vi "tmp.vi"(11 "XYGraph Refnum":refnum<vi>) -> (2 "resulting string":string)   [LabVIEW 2014, in "Graph.lvclass"]
uses:
  Graph.lvclass
  <vilib>/Analysis/1siggen.llb/Ramp Pattern by Samples.vi
  <userlib>/_OpenG.lib/array/array.llb/Remove Duplicates from 1D Array (U32)__ogtk.vi
  <userlib>/_OpenG.lib/array/array.llb/Delete Elements from 1D Array (String)__ogtk.vi
  <vilib>/gmath/NI_Gmath.lvlib
  <vilib>/Analysis/NI_AALBase.lvlib
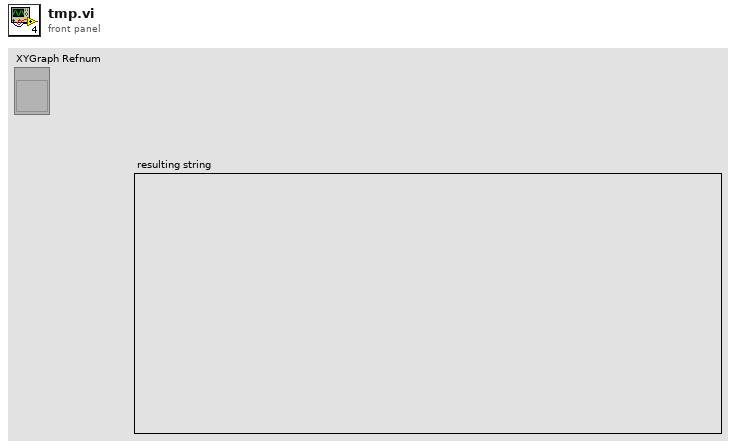
[diagram p1: front panel]
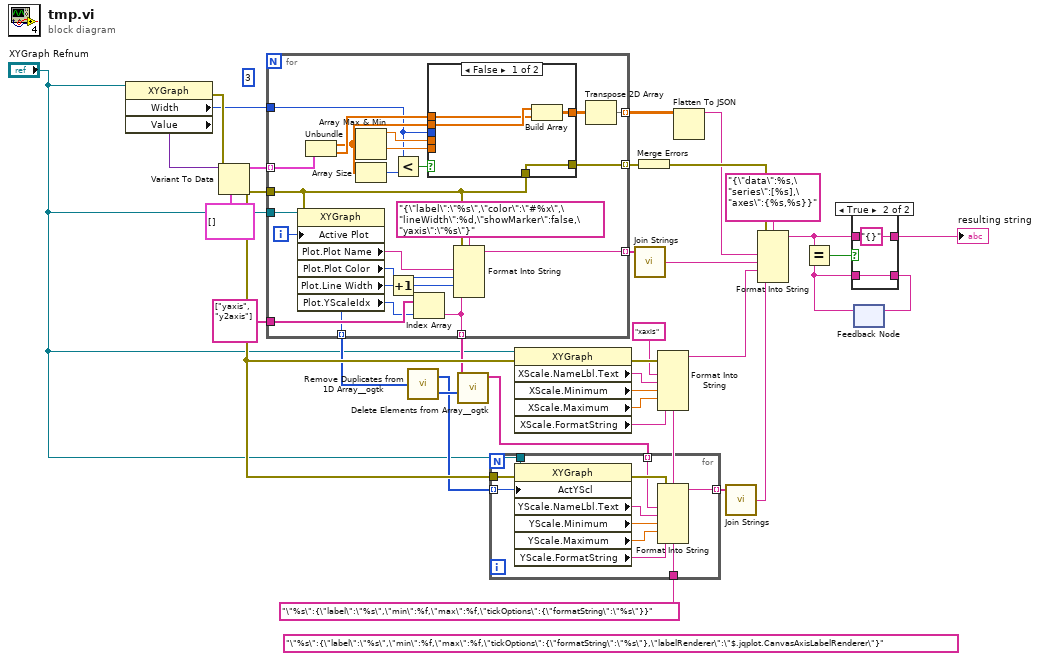
[diagram p0: block diagram]
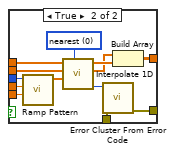
[diagram p3: hidden frame]
diagram:
  (unwired) "\"%s\":{\"label\":\"%s\",\"min\":%f,\"max\":%f,\"tickOptions\":{\"formatString\":\"%s\"},\"labelRenderer\":\"$.jqplot.CanvasAxisLabelRenderer\"}"
  (unwired) 3
  w7 = "\"%s\":{\"label\":\"%s\",\"min\":%f,\"max\":%f,\"tickOptions\":{\"formatString\":\"%s\"}}"
  n1 = property class="XYGraph"(reference="XYGraph Refnum") -> (error out=w35:errorcluster, "Width"=w6:u32, "Value"=w31:variant)  [unwired: 1 in, 1 out]
  n2 = Variant To Data(error in=w35, type=cluster{dbl[], dbl[]}[] [], Variant=w31) -> (data=w29:cluster{dbl[], dbl[]}[], error out=w34:errorcluster)
  n3 = for {
    tunnel: [w56] -> w9 mode=indexing
    tunnel: w29 -> [w53] mode=indexing
    tunnel: "XYGraph Refnum" -> [w40]
    tunnel: [w58] -> w28 mode=indexing
    tunnel: w6 -> [w47]
    tunnel: w34 -> [w57]
    tunnel: string[] ["yaxis", "y2axis"] -> [w41]
    tunnel: [w39] -> w13 mode=indexing
    tunnel: [w38] -> w12 mode=indexing
    tunnel: [w37] -> w11 mode=indexing
    i -> [w42]
    n4 = property on="Property Node" class="XYGraph"(reference=w40, error in=w57, "Active Plot"=w42) -> ("Plot.Plot Name"=w44:string, "Plot.Plot Color"=w45:u32, "Plot.Line Width"=w46:u8, "Plot.YScaleIdx"=w39:u32)  [unwired: 2 out]
    n5 = Unbundle(w53) -> (w49:dbl[], w54:dbl[])
    n6 = Array Max & Min(array=w49) -> (max value=w52:dbl, min value=w51:dbl)  [unwired: 2 out]
    n7 = Array Size(array=w49) -> (size(s)=w48:i32)
    n8 = Increment(x=w46) -> (x+1=w36:u8)
    n9 = Less?(x=w47, y=w48) -> (x < y?=w50:bool)
    n10 = Index Array(array=w41, index=w39) -> (element=w38:string)
    n11 = case shown="False" w50 {
      tunnel: [w59 w75] -> w58
      tunnel: [w62 w73] -> w55
      tunnel: w54 -> [w60 w72]
      tunnel: w49 -> [w61 w66]
      tunnel: w52 -> [_ w65]
      tunnel: w51 -> [_ w64]
      tunnel: w47 -> [_ w63]
      tunnel: w57 -> [w59 w74]
      frame False {
        n12 = Build Array(w61, w60) -> (w62:dbl[][])
      }
      frame True {
        w67 = 0 items=["nearest", "linear", "spline", "cubic Hermite", "Lagrange"] ("method")
        n13 = call-poly <vilib>:"Ramp Pattern.vi"("start"=w64, "end"=w65, "samples"=w63) -> ("Ramp Pattern"=w68:dbl[])  [unwired: 7 in, 1 out]
        n14 = call <vilib>:"Interpolate 1D.vi"("method"=w67, "xi"=w68, "X"=w66, "Y"=w72) -> ("error"=w69:i32, "xi used"=w70:dbl[], "yi"=w71:dbl[])  [unwired: 5 in]
        n15 = call <vilib>:"Error Cluster From Error Code.vi"("error in (no error)"=w74, "error code (0)"=w69) -> ("error out"=w75:errorcluster)  [unwired: 7 in]
        n16 = Build Array(w70, w71) -> (w73:dbl[][])
      }
    }
    n17 = Format Into String(format string="{\"label\":\"%s\",\"color\":\"#%x\",\"lineWidth\":%d,\"showMarker\":false,\"yaxis\":\"%s\"}", error in=w57, w44, w45, w36, w38) -> (resulting string=w37:string)  [unwired: 1 in, 1 out]
    n18 = Transpose 2D Array(2D array=w55) -> (transposed array=w56:dbl[][])
  }
  n19 = call-poly <userlib>:"Remove Duplicates from 1D Array__ogtk.vi"("Input Array"=w13) -> ("Output Array"=w14:u32[], "indices of removed elements"=w25:i32[])
  n20 = call-poly <userlib>:"Delete Elements from Array__ogtk.vi"("indices"=w25, "array"=w12) -> ("array w/ subset deleted"=w26:string[])  [unwired: 8 in, 1 out]
  n21 = for {
    tunnel: w14 -> [w84] mode=indexing
    tunnel: w26 -> [w82] mode=indexing
    tunnel: [w78] -> w15 mode=indexing
    tunnel: w7 -> [w77]
    tunnel: "XYGraph Refnum" -> [w76]
    tunnel: w34 -> [w86]
    n22 = property on="Property Node" class="XYGraph"(reference=w76, error in=w86, "ActYScl"=w84) -> (error out=w85:errorcluster, "YScale.NameLbl.Text"=w83:string, "YScale.Minimum"=w81:dbl, "YScale.Maximum"=w80:dbl, "YScale.FormatString"=w79:string)  [unwired: 1 out]
    n23 = Format Into String(format string=w77, error in=w85, w82, w83, w81, w80, w79) -> (resulting string=w78:string)  [unwired: 1 in, 1 out]
  }
  n24 = property on="Property Node" class="XYGraph"(reference="XYGraph Refnum", error in=w34) -> (error out=w33:errorcluster, "XScale.NameLbl.Text"=w19:string, "XScale.Minimum"=w20:dbl, "XScale.Maximum"=w21:dbl, "XScale.FormatString"=w22:string)  [unwired: 1 out]
  n25 = call <vilib>:"Join Strings.vi"("Strings In"=w11) -> ("String"=w18:string)  [unwired: 2 in]
  n26 = Merge Errors(w28) -> (w32:errorcluster)
  n27 = Format Into String(format string=w7, error in=w33, "xaxis", w19, w20, w21, w22) -> (resulting string=w23:string)  [unwired: 1 in, 1 out]
  n28 = Flatten To JSON(anything=w9) -> (JSON string=w8:string)  [unwired: 2 in, 1 out]
  n29 = call <vilib>:"Join Strings.vi"("Strings In"=w15) -> ("String"=w17:string)  [unwired: 2 in]
  n30 = Format Into String(format string="{\"data\":%s,\"series\":[%s],\"axes\":{%s,%s}}", error in=w32, w8, w18, w23, w17) -> (resulting string=w2:string)  [unwired: 1 in, 1 out]
  n31 = feedback #1() -> (w3:string)  [unwired: 1 in]
  n32 = Equal?(x=w2, y=w3) -> (x = y?=w5:bool)
  n33 = case shown="True" w5 {
    tunnel: [w87 w89] -> w4
    tunnel: w3 -> [_ w89]
    tunnel: w2 -> [w87 _]
    tunnel: [w87 "{}"] -> w1
    frame False {
    }
    frame True {
    }
  }
  "resulting string" <- w1
  n34 = feedback-in #1(w4) -> ()
